vi "FPGA Debounce Filter Multichannel.vi"(5 "Channel #":u32, 8 "Debounce (iterations)":i32=1, 9 "Input":bool) -> (2 "Output[k-1]":bool, 3 "Output":bool)   [LabVIEW 2015]
uses:
  <vilib>/rvi/DataTransferAndStorage/Container/Common/niFpgaContainerGetUniqueNameForEmu.vi
  <vilib>/rvi/DataTransferAndStorage/Container/Common/niFpgaContainerSetEmuInfo.vi
  <vilib>/rvi/eio/common/nirviEmuReportErrorAndStop.vi
  <vilib>/rvi/DataTransferAndStorage/Container/Common/niFpgaContainerExecOnDevCompGetState.vi
  <vilib>/rvi/Emulation/niFpgaEmulationIsFPGAContextNoSignature.vi
  <vilib>/rvi/Emulation/niFpgaProcessEmulError.vi
  <vilib>/rvi/Emulation/niFpgaSctlEmulationGetInTimedLoop.vi
  <vilib>/rvi/errors/nirviReportUnexpectedCaseInternalError (U32).vi
  <vilib>/rvi/Memory/Memory_Emulation/niFpgaMemoryEmulationCacheClearOnFirstRun.vi
  <vilib>/rvi/Memory/Memory_Emulation/nirvimemoryEmulationManagerCache_MakeExclusive.vi
  <vilib>/rvi/Memory/Memory_Emulation/niFpgaMemoryEmulationValidateCache.vi
  <vilib>/rvi/Memory/Memory_Emulation/nirvimemoryEmulationManagerCache_InsertValue.vi
  <vilib>/Utility/error.llb/Clear Errors.vi
  <vilib>/rvi/Memory/Memory_Emulation/nirvimemoryEmulationManagerCache_ReleaseExclusive.vi
  <vilib>/rvi/Memory/Memory_Emulation/nirvimemoryEmulationManagerCache_GetValue.vi
  <vilib>/rvi/Memory/Memory_Emulation/nirvimemoryEmulationManagerCache_SetValue.vi
  <vilib>/rvi/Emulation/niFpgaSctlEmulationResourceMgr.vi
  <vilib>/rvi/LocalResourceManager/LocalResourceManager.xnode
  <vilib>/rvi/DataTransferAndStorage/Container/XNode/niFpgaContainer.xnode
  <vilib>/rvi/Memory/Memory_Emulation/niFpgaMemoryEmulationRefIn.vi
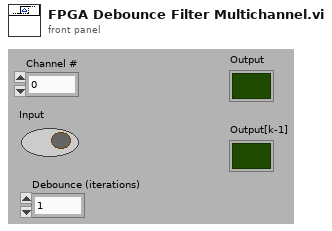
[diagram p1: front panel]
types:
  T1 = cluster{"Input[k-1]":bool, "Counter":i32, "Output[k-1]":bool}
  T2 = cluster{"Input":bool, "Counter":i32, "Input":bool}
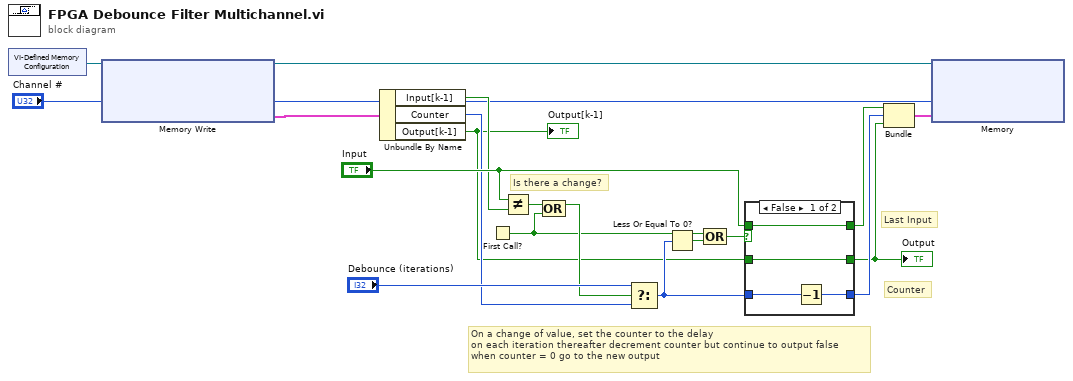
[diagram p0: block diagram]
diagram:
  # "Counter"
  # "Last Input"
  # "Is there a change?"
  # "On a change of value, set the counter to the delay\non each iteration thereafter decrement counter but continue to output false\nwhen counter = 0 go to the new output"
  n1 = xnode ("VI-Defined Memory Configuration")() -> ("Memory Out"=w5:refnum<k21>)
  n2 = xnode "Memory Write"("Address"="Channel #", "Memory In"=w5) -> ("Data"=w4:T1, "Memory Out"=w3:refnum<k21>)
  n3 = Unbundle By Name(w4) -> ("Input[k-1]"=w11:bool, "Counter"=w8:i32, "Output[k-1]"=w6:bool)
  "Output[k-1]" <- w6
  n4 = First Call?() -> (First Call?: T/F=w13:bool)
  n5 = Not Equal?(x="Input", y=w11) -> (x != y?=w16:bool)
  n6 = Compound Arithmetic op=OR(w16, w13) -> (w15:bool)
  n7 = Select(t="Debounce (iterations)", s=w15, f=w8) -> (s? t:f=w18:i32)
  n8 = Less Or Equal To 0?(x=w18) -> (x <= 0?=w14:bool)
  n9 = Compound Arithmetic op=OR(w13, w14) -> (w12:bool)
  n10 = case shown="False" w12 {
    tunnel: [w20 w24] -> w7
    tunnel: "Input" -> [w21 w24]
    tunnel: w18 -> [w23 w25]
    tunnel: [w22 w25] -> w9
    tunnel: [w21 w24] -> w10
    tunnel: w6 -> [w20 _]
    frame False {
      n11 = Decrement(x=w23) -> (x-1=w22:i32)
    }
    frame True {
    }
  }
  "Output" <- w7
  n12 = Bundle("Input"=w10, "Counter"=w9, "Input"=w7) -> (w1:T2)  [unwired: 1 in]
  n13 = xnode "Memory"("Address"="Channel #", "Data"=w1, "Memory In"=w3) -> ()  [unwired: 1 out]
